vi "GetDataVersion.vi"(0 "session In":refnum<k35>, 5 "GEA2 Reference In":refnum<k24>, 11 "error In":errorcluster) -> (4 "session out":refnum<k35>, 8 "Data Version Out":cluster{"ERD Number":u16, "Data":string}[](array[cluster]), 15 "error out":errorcluster)   [LabVIEW 2021]
uses:
  D:/Common/LabVIEW GEA2 Toolkit/source/GEA3 DLL Source/GeaCommunication.dll
  Common/LabVIEW GEA2 Toolkit/source/GEA3 DLL Source/GeaCommunication.dll
  Common/LabVIEW GEA2 Toolkit/GEA3/type defs/Data Type.ctl
  Common/LabVIEW GEA2 Toolkit/GEA3/library/GEA2_Toolkit.lvlib
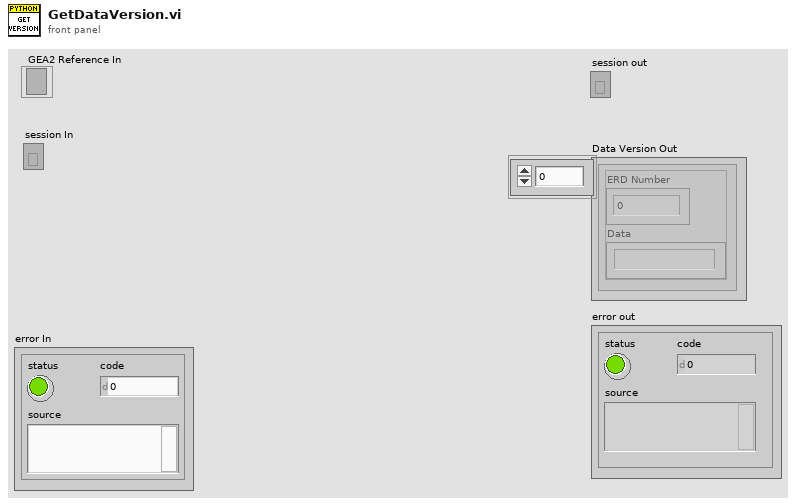
[diagram p1: front panel]
types:
  T1 = typedef "Data Type.ctl" = enum16{"string", "boolean", "uint8_t", "uint16_t", "uint32_t", "uint64_t", "int8_t", "int16_t", "int32_t", "int64_t"}
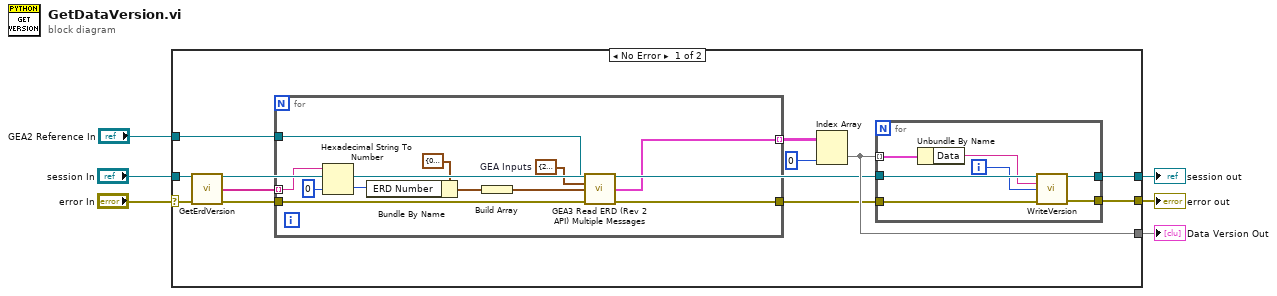
[diagram p0: block diagram]
diagram:
  n1 = case shown="No Error" "error In" {
    selector: "error In" -> [w8 w38]
    tunnel: [w15 _] -> w1
    tunnel: "GEA2 Reference In" -> [w11 _]
    tunnel: "session In" -> [w10 w37]
    tunnel: [w9 w37] -> w3
    tunnel: [w7 w38] -> w2
    frame No Error {
      n2 = call "GetErdVersion.vi"("session in"=w10, "error In"=w8) -> ("session Out"=w14:refnum<k35>, "Erds To Read"=w18:string[], "error Out"=w13:errorcluster)  [unwired: 11 in]
      n3 = for {
        tunnel: w11 -> [w36]
        tunnel: w13 -> [w35]
        tunnel: w18 -> [w30] mode=indexing
        tunnel: [w28] -> w17 mode=indexing
        tunnel: [w27] -> w12
        w34 = cluster{"Source":u8, "Destination":u8} {"Source"=229, "Destination"=192}  # GEA Inputs
        n4 = Hexadecimal String To Number(string=w30, default (0uL)=u16 0 ("ERD Number")) -> (number=w29:u16)  [unwired: 1 in, 1 out]
        n5 = Bundle By Name(cluster=cluster{"ERD Number":u16, "Data Type":T1} {"ERD Number"=0, "Data Type"=enum."string"} ("ERD Read Data In"), "ERD Number"=w29) -> (w33:cluster{"ERD Number":u16, "Data Type":T1})
        n6 = Build Array(w33) -> (w31:cluster{"ERD Number":u16, "Data Type":T1}[])
        n7 = call "GEA3 Read ERD (Rev 2 API) Multiple Messages.vi"("GEA2 Reference In"=w36, "GEA Inputs"=w34, "Read ERD List"=w31, "Error In"=w35) -> ("ERD Data Out"=w28:cluster{"ERD Number":u16, "Data":string}[], "Error Out"=w27:errorcluster)  [unwired: 8 in, 2 out]
      }
      n8 = Index Array(array=w17, index (col)=0 ("disabled index (col)")) -> (element=w15:cluster{"ERD Number":u16, "Data":string}[])  [unwired: 1 in]
      n9 = for {
        tunnel: w15 -> [w25] mode=indexing
        tunnel: w14 -> [w23]
        tunnel: [w24] -> w9
        tunnel: w12 -> [w22]
        tunnel: [w19] -> w7
        i -> [w20]
        n10 = Unbundle By Name(w25) -> ("Data"=w21:string)
        n11 = call "WriteVersion.vi"("session in"=w23, "Data input"=w21, "index"=w20, "error In"=w22) -> ("session out"=w24:refnum<k35>, "error Out"=w19:errorcluster)  [unwired: 10 in]
      }
    }
    frame Error {
    }
  }
  "session out" <- w3
  "error out" <- w2
  "Data Version Out" <- w1
